vi "FTW-JSON-Core-GetRootObject.vi"(0 "JSON Object":refnum<class "FTW-JSON.lvclass">, 11 "error in":errorcluster) -> (4 "JSON Object out":refnum<class "FTW-JSON.lvclass">, 6 "JSON Library Filepath":path, 8 "JSON Object":i64 format="%016x", 15 "error out":errorcluster)   [LabVIEW 2013, in "FTW-JSON.lvclass"]
uses:
  FTW-JSON.lvclass
  FTW-JSON.lvclass/FTW-JSON.ctl
  error/FTW-ERR-ThrowGenericError.vi
  error/FTW-ERR-ThrowError.vi
  error/FTW-ERR-NoErrorConstant.vi
  error/FTW-ERR-CallChain.vi
  string/FTW-STR-ReplaceWhitespace.vi
panel:
  # "Inputs"
  # "Outputs"
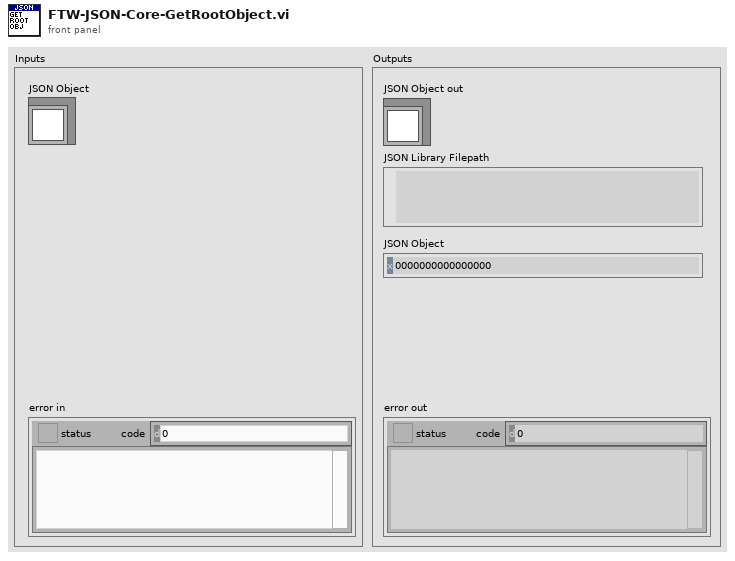
[diagram p1: front panel]
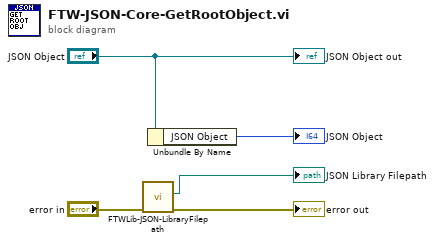
[diagram p0: block diagram]
diagram:
  n1 = call "FTWLib-JSON-LibraryFilepath.vi"("error in"="error in") -> ("error out"=→"error out":errorcluster, "JSON Library Filepath"=→"JSON Library Filepath":path)  [unwired: 9 in]
  n2 = Unbundle By Name("JSON Object") -> ("JSON Object"=→"JSON Object":i64)
  "JSON Object out" <- "JSON Object"
